vi "ASCII 읽기.vi"() -> ()   [LabVIEW 2014]
panel:
  out "웨이브폼 그래프":dbl[][](graph)
  out "텍스트":string
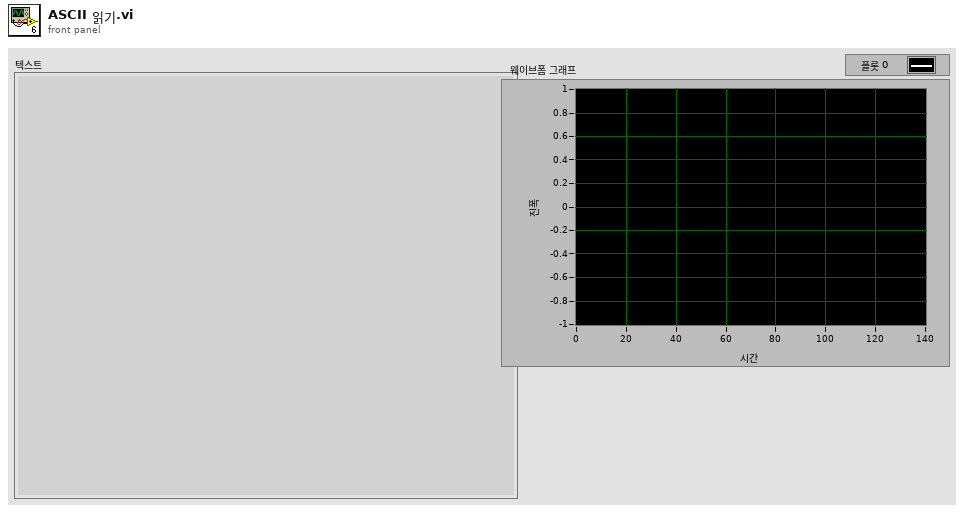
[diagram p1: front panel]
types:
  T1 = enum16{"open", "replace", "create", "open or create", "replace or create", "replace or create with confirmation"}
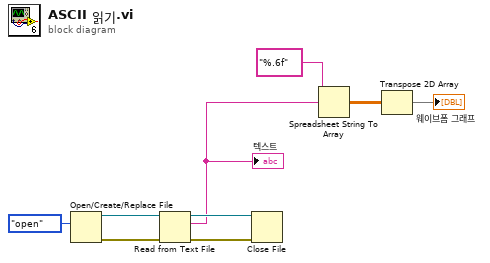
[diagram p0: block diagram]
diagram:
  n1 = Open/Create/Replace File(operation (0:open)=T1."open" ("동작(0:open)")) -> (refnum out=w8:refnum<file>, error out=w6:errorcluster)  [unwired: 5 in, 1 out]
  n2 = Read from Text File(file (use dialog)=w8, error in=w6) -> (refnum out=w7:refnum<file>, text=w4:string, error out=w5:errorcluster)  [unwired: 2 in, 1 out]
  "텍스트" <- w4
  n3 = Close File(refnum=w7, error in=w5) -> ()  [unwired: 2 out]
  n4 = Spreadsheet String To Array(format string="%.6f" ("포맷 문자열"), spreadsheet string=w4) -> (array=w2:dbl[][])  [unwired: 2 in]
  n5 = Transpose 2D Array(2D array=w2) -> (transposed array=→"웨이브폼 그래프":dbl[][])
